vi "Main.vi"() -> ()   [LabVIEW 2019]
uses:
  Shared/Controls/Intake States.ctl
  Controls/Configurator Data.ctl
  Motion Profile Trapezoid Generator/API/Motion Profile Generator/Type Defs/Motion Profile Point.ctl
  Controls/Configurator States.ctl
  Motion Profile Trapezoid Generator/API/Motion Profile Generator/Type Defs/Control Boundaries.ctl
  Motion Profile Trapezoid Generator/API/Motion Profile Generator/Motion Profile Generator.lvclass/Motion Profile Generator.ctl
  Motion Profile Trapezoid Generator/API/Motion Profile Generator/Public Methods/Read Motion Profile Array.vi
  <vilib>/Utility/file.llb/Write Delimited Spreadsheet (string).vi
  Motion Profile Trapezoid Generator/API/Motion Profile Generator/Motion Profile Generator.lvclass
panel:
  out "File":string[][](array[string])
  out "Plot":cluster{dbl[], dbl[]}[](graph)
  out "Cluster":T1
  in  "Status":T4={"Intake"=[{"State"=enum."Retracted", "Absolute time (s)"=0.0}, {"State"=enum."Extended", "Absolute time (s)"=0.1}, {"State"=enum."Extended", "Absolute time (s)"=0.5}, {"State"=enum."Retracted", "Absolute time (s)"=0.0}, {"State"=enum."Extended", "Absolute time (s)"=2.0}, {"State"=enum."Retracted", "Absolute time (s)"=4.0}, {"State"=enum."Extended", "Absolute time (s)"=6.0}, {"State"=enum."Retracted", "Absolute time (s)"=8.0}, {"State"=enum."Extended", "Absolute time (s)"=8.2}]}
  in  "Time Between Points (ms)":dbl=20.0
  in  "Generate MP":bool
  in  "Create File":bool
  in  "Stop":bool
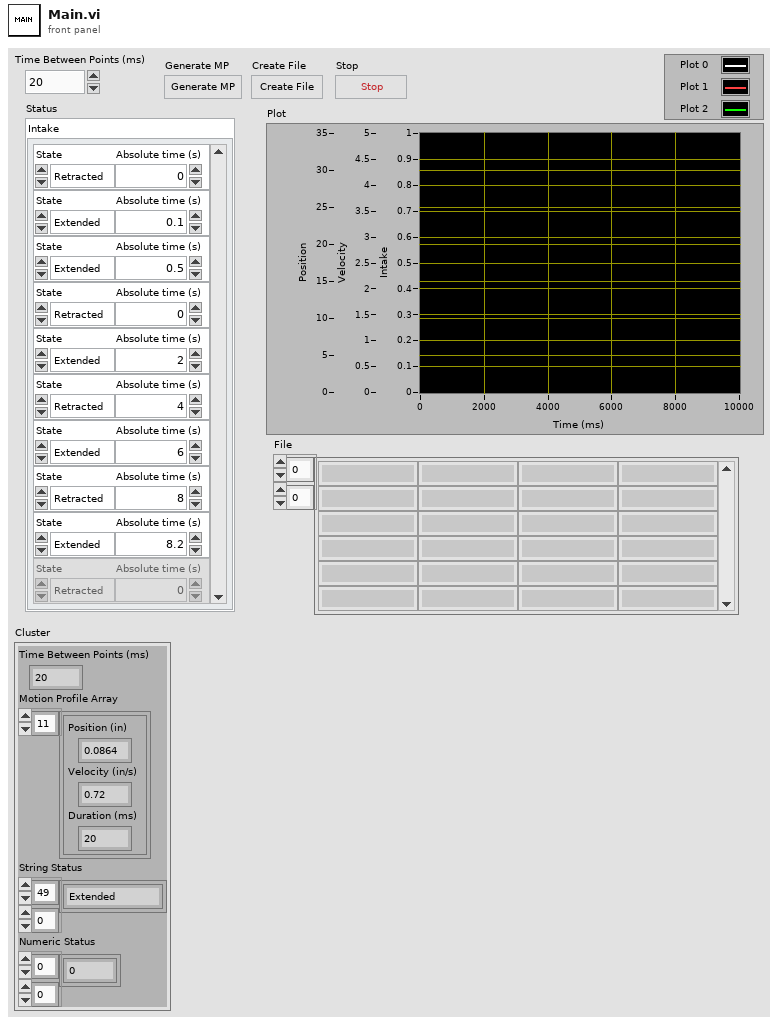
[diagram p1: front panel]
types:
  T1 = typedef "Configurator Data.ctl" = cluster{"Time Between Points (ms)":dbl, "Motion Profile Array":T2[], "String Status":string[][], "Numeric Status":i32[][]}
  T2 = typedef "Motion Profile Generator.lvclass/Motion Profile Point.ctl" = cluster{"Position (in)":dbl, "Velocity (in/s)":dbl, "Duration (ms)":dbl}
  T3 = typedef "Intake States.ctl" = enum16{"Retracted", "Extended"}
  T4 = cluster{"Intake":cluster{"State":T3, "Absolute time (s)":dbl}[]}
  T5 = typedef "Configurator States.ctl" = enum16{"Initialize", "Wait for Event", "Create File"}
  T6 = typedef "Motion Profile Generator.lvclass/Control Boundaries.ctl" = cluster{"Max Speed (in/s)":dbl, "Max Acceleration (in/s2)":dbl, "Max Deceleration (in/s2)":dbl}
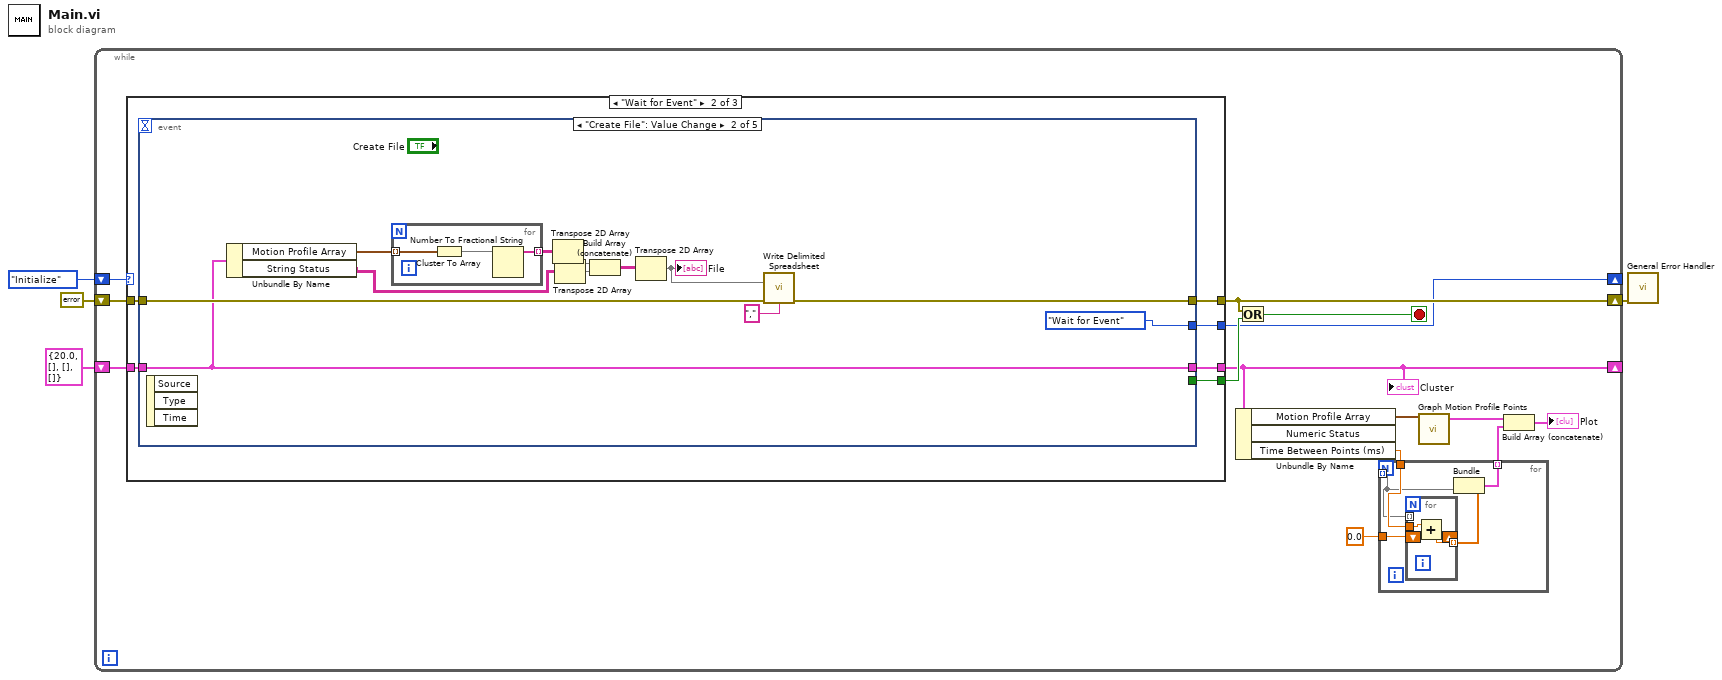
[diagram p0: block diagram]
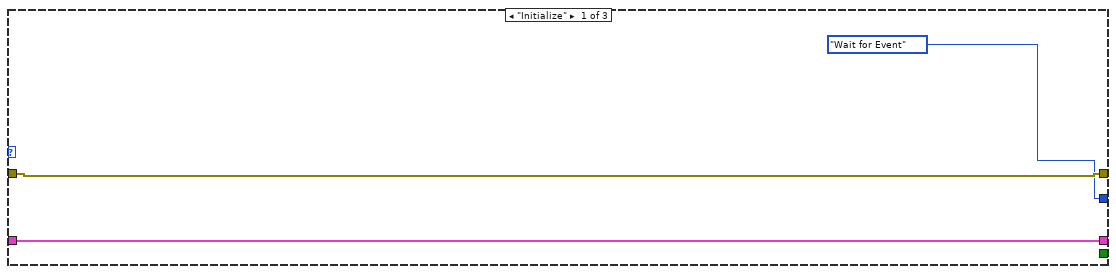
[diagram p2: hidden frame]
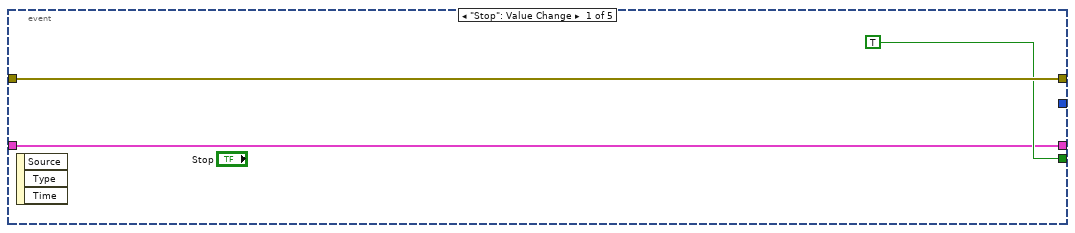
[diagram p3: hidden frame]
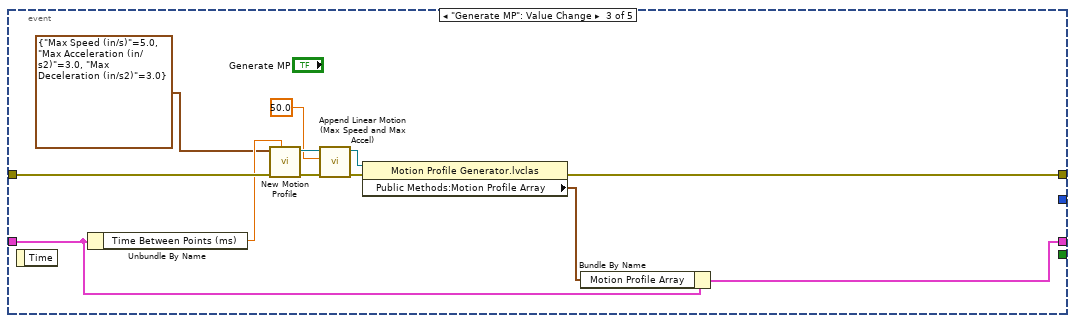
[diagram p4: hidden frame]
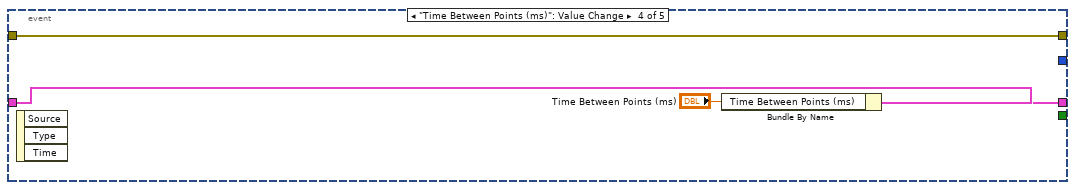
[diagram p5: hidden frame]
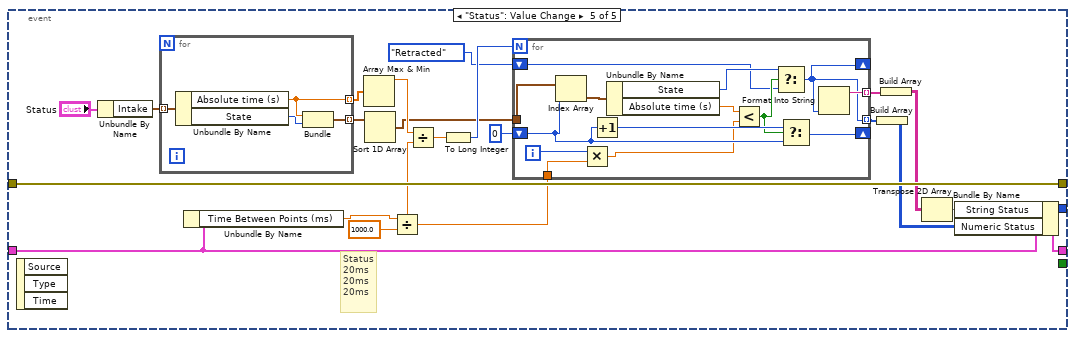
[diagram p6: hidden frame]
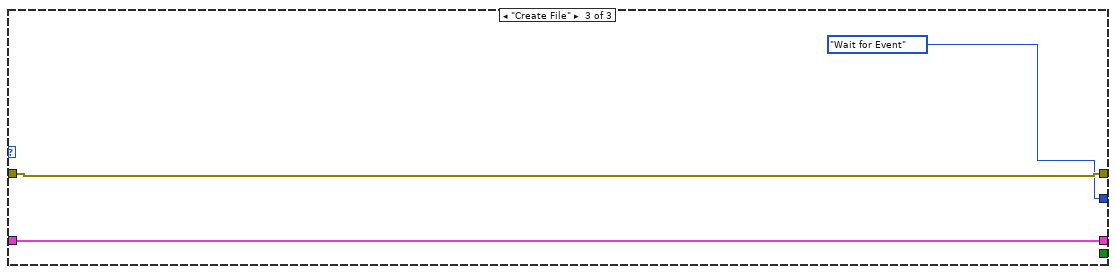
[diagram p7: hidden frame]
diagram:
  n1 = while {
    shift-right: [w13] -> _
    shift-left: Configurator_States."Initialize" ("Configurator States") -> [w19]
    shift-right: [w16] -> w2
    shift-left: errorcluster {"status"=FALSE, "code"=0, "source"=""} ("error constant") -> [w18]
    shift-right: [w12] -> _
    shift-left: T1 {"Time Between Points (ms)"=20.0, "Motion Profile Array"=[], "String Status"=[], "Numeric Status"=[]} -> [w14]
    stop <- w17 stop-if-true
    n2 = case shown="\"Wait for Event\"" w19 {
      tunnel: [w30 w36 w112] -> w16
      tunnel: w18 -> [w30 w35 w112]
      tunnel: [_ w34 _] -> w15
      tunnel: [w29 w33 w111] -> w12
      tunnel: w14 -> [w29 w32 w111]
      tunnel: [Configurator_States."Wait for Event" ("Configurator States") w31 Configurator_States."Wait for Event" ("Configurator States")] -> w13
      frame "Initialize" {
      }
      frame "Wait for Event" {
        n3 = event shown="[1] \"Create File\": Value Change" {
          selector: _ -> [_ _ _ _ _]
          dyn-events: _ -> [_ _ _ _ _]
          timeout: _ -> [_ _ _ _ _]
          tunnel: [w39 w42 w60 w70 w91] -> w36
          tunnel: w35 -> [w39 w51 w66 w70 w91]
          tunnel: [TRUE _ _ _ _] -> w34
          tunnel: [w37 w49 w58 w68 w90] -> w33
          tunnel: w32 -> [w37 w49 w62 w69 w87]
          tunnel: [_ Configurator_States."Wait for Event" ("Configurator States") _ _ _] -> w31
          event "Stop": Value Change {
            n4 = event-data() -> ()  [unwired: 1 in, 3 out]
          }
          event "Create File": Value Change {
            n5 = event-data() -> ()  [unwired: 1 in, 3 out]
            n6 = Unbundle By Name(w49) -> ("Motion Profile Array"=w48:T2[], "String Status"=w46:string[][])
            n7 = for {
              tunnel: w48 -> [w54] mode=indexing
              tunnel: [w52] -> w47 mode=indexing
              n8 = Cluster To Array(cluster=w54) -> (array=w53:dbl[])
              n9 = Number To Fractional String(number=w53) -> (F-format string=w52:string[])  [unwired: 3 in]
            }
            n10 = Transpose 2D Array(2D array=w47) -> (transposed array=w45:string[][])
            n11 = Transpose 2D Array(2D array=w46) -> (transposed array=w44:string[][])
            n12 = Build Array (concatenate)(w45, w44) -> (w43:string[][])
            n13 = Transpose 2D Array(2D array=w43) -> (transposed array=w41:string[][])
            "File" <- w41
            n14 = call-poly <vilib>:"Write Delimited Spreadsheet.vi"("2D data"=w41, "error in (no error)"=w51, "delimiter (\\t)"="," ("delimiter (\\t)")) -> ("error out"=w42:errorcluster)  [unwired: 11 in, 1 out]
          }
          event "Generate MP": Value Change {
            n15 = event-data() -> ()  [unwired: 1 in, 1 out]
            n16 = Unbundle By Name(w62) -> ("Time Between Points (ms)"=w61:dbl)
            n17 = call "New Motion Profile.vi"("Time Between Points (ms)"=w61, "error in (no error)"=w66, "Control Boundaries"=T6 {"Max Speed (in/s)"=5.0, "Max Acceleration (in/s2)"=3.0, "Max Deceleration (in/s2)"=3.0}) -> ("error out"=w64:errorcluster, "Motion Profile Generator out"=w65:refnum<class "Motion Profile Generator.lvclass">)  [unwired: 7 in]
            n18 = call "Append Linear Motion (Max Speed and Max Accel).vi"("error in (no error)"=w64, "Distance (in)"=50.0, "Motion Profile Generator in"=w65) -> ("error out"=w63:errorcluster, "Motion Profile Generator out"=w59:refnum<class "Motion Profile Generator.lvclass">)  [unwired: 7 in]
            n19 = property class="Motion Profile Generator.lvclas"(reference=w59, error in=w63) -> (error out=w60:errorcluster, "Public Methods:Motion Profile Array"=w57:T2[])  [unwired: 1 out]
            n20 = Bundle By Name(cluster=w62, "Motion Profile Array"=w57) -> (w58:T1)
          }
          event "Time Between Points (ms)": Value Change {
            n21 = event-data() -> ()  [unwired: 1 in, 3 out]
            n22 = Bundle By Name(cluster=w69, "Time Between Points (ms)"="Time Between Points (ms)") -> (w68:T1)
          }
          event "Status": Value Change {
            # "Status\n20ms\n20ms\n20ms"
            n23 = event-data() -> ()  [unwired: 1 in, 3 out]
            n24 = Unbundle By Name("Status") -> ("Intake"=w88:cluster{"State":T3, "Absolute time (s)":dbl}[])
            n25 = for {
              tunnel: w88 -> [w109] mode=indexing
              tunnel: [w108] -> w86 mode=indexing
              tunnel: [w106] -> w80 mode=indexing
              n26 = Unbundle By Name(w109) -> ("Absolute time (s)"=w108:dbl, "State"=w107:T3)
              n27 = Bundle("Absolute time (s)"=w108, "State"=w107) -> (w106:cluster{"Absolute time (s)":dbl, "State":T3})  [unwired: 1 in]
            }
            n28 = Unbundle By Name(w87) -> ("Time Between Points (ms)"=w85:dbl)
            n29 = Array Max & Min(array=w86) -> (max value=w83:dbl)  [unwired: 3 out]
            n30 = Sort 1D Array(array=w80) -> (sorted array=w79:cluster{"Absolute time (s)":dbl, "State":T3}[])
            n31 = Divide(x=w85, y=1000.0) -> (x/y=w77:dbl)
            n32 = Divide(x=w83, y=w77) -> (x/y=w82:dbl)
            n33 = To Long Integer(number=w82) -> (32bit integer=w81:i32)
            n34 = for {
              N: w81 -> [_]
              tunnel: w79 -> [w105]
              shift-right: [w104] -> _
              shift-left: 0 -> [w102]
              tunnel: w77 -> [w98]
              shift-right: [w92] -> _
              shift-left: Intake_States."Retracted" ("State") -> [w94]
              tunnel: [w93] -> w73 mode=indexing
              tunnel: [w92] -> w72 mode=indexing
              i -> [w99]
              n35 = Index Array(array=w105, index=w102) -> (element=w101:cluster{"Absolute time (s)":dbl, "State":T3})
              n36 = Multiply(x=w99, y=w98) -> (x*y=w97:dbl)
              n37 = Increment(x=w102) -> (x+1=w103:i32)
              n38 = Unbundle By Name(w101) -> ("State"=w95:T3, "Absolute time (s)"=w100:dbl)
              n39 = Less?(x=w100, y=w97) -> (x < y?=w96:bool)
              n40 = Select(t=w95, s=w96, f=w94) -> (s? t:f=w92:T3)
              n41 = Select(t=w103, s=w96, f=w102) -> (s? t:f=w104:i32)
              n42 = Format Into String(w92) -> (resulting string=w93:string)  [unwired: 3 in, 1 out]
            }
            n43 = Build Array(w72) -> (w71:T3[][])
            n44 = Build Array(w73) -> (w75:string[][])
            n45 = Transpose 2D Array(2D array=w75) -> (transposed array=w74:string[][])
            n46 = Bundle By Name(cluster=w87, "String Status"=w74, "Numeric Status"=w71) -> (w90:T1)
          }
        }
      }
      frame "Create File" {
      }
    }
    "Cluster" <- w12
    n47 = Unbundle By Name(w12) -> ("Motion Profile Array"=w11:T2[], "Numeric Status"=w8:i32[][], "Time Between Points (ms)"=w5:dbl)
    n48 = Or(x=w16, y=w15) -> (x .or. y?=w17:bool)
    n49 = for {
      tunnel: w8 -> [w20] mode=indexing
      tunnel: [w23] -> w7 mode=indexing
      tunnel: 0.0 -> [w22]
      tunnel: w5 -> [w21]
      n50 = for {
        tunnel: [w25] -> w24 mode=indexing
        tunnel: w21 -> [w26]
        tunnel: w20 -> [_] mode=indexing
        shift-right: [w25] -> _
        shift-left: w22 -> [w27]
        n51 = Add(x=w26, y=w27) -> (x+y=w25:dbl)
      }
      n52 = Bundle(w24, "Numeric Status"=w20) -> (w23:cluster{dbl[], "Numeric Status":i32[]})  [unwired: 1 in]
    }
    n53 = call "Graph Motion Profile Points.vi"("Motion Profile Array"=w11) -> ("Array"=w10:cluster{dbl[], dbl[]}[])  [unwired: 10 in]
    n54 = Build Array (concatenate)(w10, w7) -> (→"Plot":cluster{dbl[], "Numeric Status":dbl[]}[])
  }
  n55 = call <vilib>:"General Error Handler.vi"("error in (no error)"=w2) -> ()  [unwired: 10 in, 5 out]
